vi "parse_search_points_response.vi"(8 "error in (no error)":errorcluster, 10 "body":string, 11 "headers":string) -> (0 "error out":errorcluster, 2 "scores":dbl[](array[numeric]), 3 "ids":string[](array[string]))   [LabVIEW 2020, in "vector_qdrant.lvclass"]
uses:
  vector_qdrant.lvclass
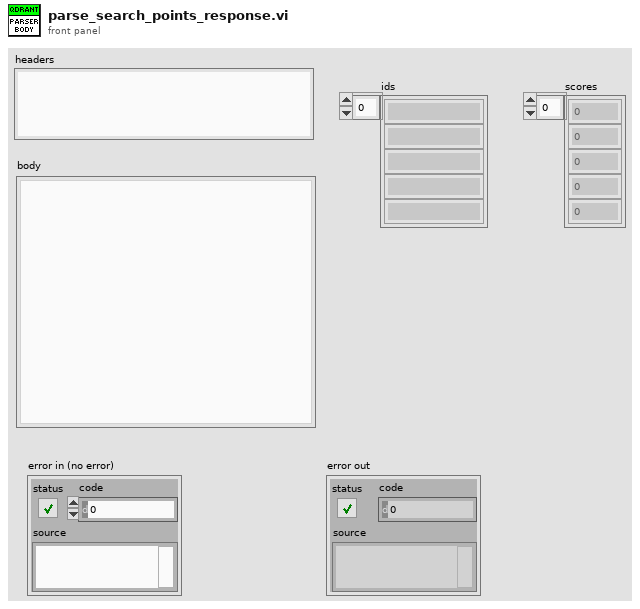
[diagram p1: front panel]
types:
  T1 = cluster{"id":string, "version":i32, "score":dbl}[]
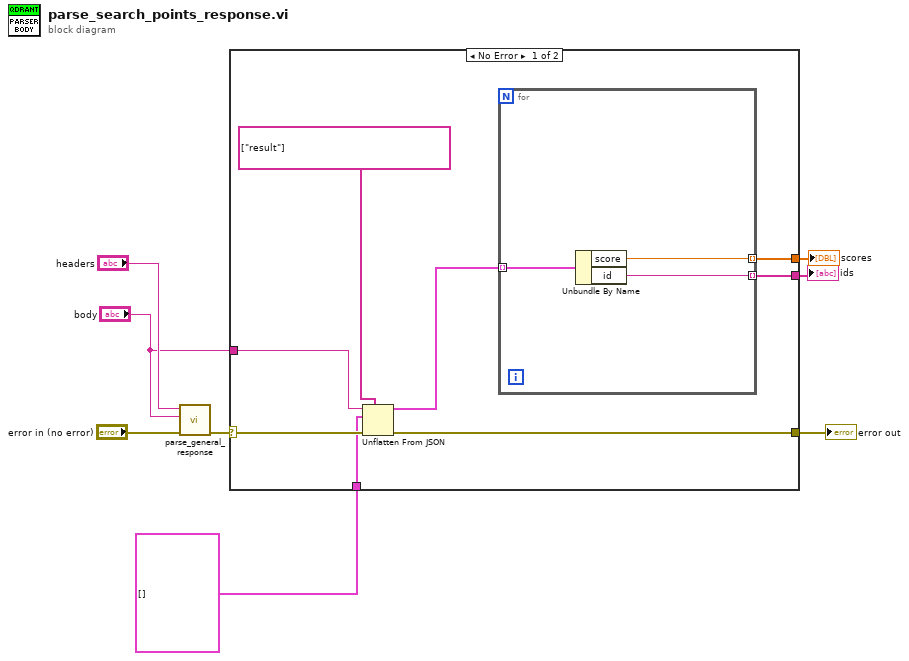
[diagram p0: block diagram]
diagram:
  n1 = call "parse_general_response.vi"("error in (no error)"="error in (no error)", "body"="body", "headers"="headers") -> ("error out"=w6:errorcluster)  [unwired: 8 in]
  n2 = case shown="No Error" w6 {
    selector: w6 -> [w16 w20]
    tunnel: [w13 w20] -> w8
    tunnel: "body" -> [w14 _]
    tunnel: T1 [] -> [w12 _]
    tunnel: [w10 _] -> w1
    tunnel: [w9 _] -> w2
    frame No Error {
      n3 = Unflatten From JSON(path=string[] ["result"], JSON string=w14, type and defaults=w12, error in (no error)=w16) -> (value=w11:T1, error out=w13:errorcluster)  [unwired: 3 in]
      n4 = for {
        tunnel: w11 -> [w19] mode=indexing
        tunnel: [w18] -> w10 mode=indexing
        tunnel: [w17] -> w9 mode=indexing
        n5 = Unbundle By Name(w19) -> ("score"=w17:dbl, "id"=w18:string)
      }
    }
    frame Error {
    }
  }
  "error out" <- w8
  "scores" <- w2
  "ids" <- w1
